vi "SetTrendPointProperties.vi"(8 "error in (no error)":errorcluster, 10 "map":T2, 11 "data set id":string) -> (0 "error out":errorcluster, 3 "properties":T1[](array[typedef]))   [LabVIEW 2017, in "IrDataEventCreator.lvlib"]
uses:
  <vilib>/addons/InsightCM/Devices/Shared/Ir/IrDataEventCreator/IrDataEventCreator.lvlib
  <vilib>/addons/PointValueMap/controls/PointMap.ctl
  <vilib>/addons/InsightCM/MessageBus/Base/controls/KeyValuePair.ctl
  <vilib>/addons/PointValueMap/subVIs/Point_Read_string.vi
  <vilib>/addons/PointValueMap/PointValueMap.lvlib
  <vilib>/addons/InsightCM/Utilities/PropertyHelpers/PropertyHelpers.lvlib
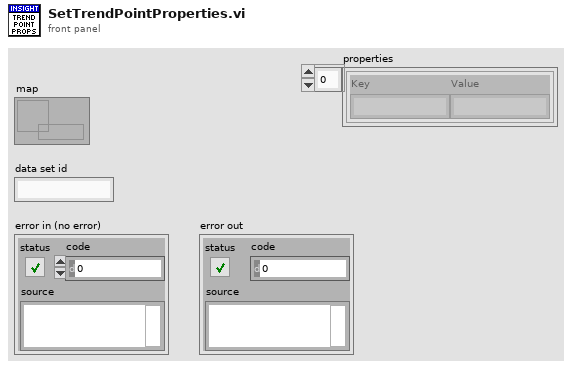
[diagram p1: front panel]
types:
  T1 = typedef "KeyValuePair.ctl" = cluster{"Key":string, "Value":string}
  T2 = typedef "PointValueMap.lvlib/PointMap.ctl" = refnum<data-value>
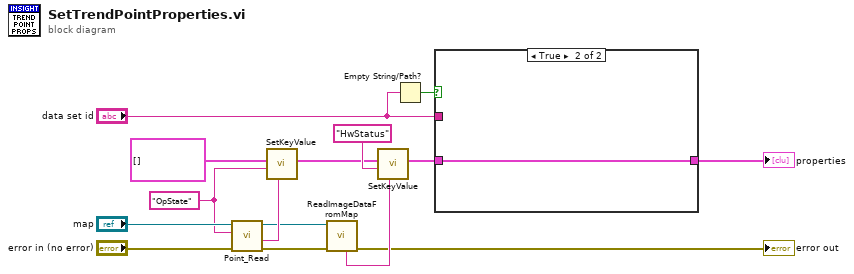
[diagram p0: block diagram]
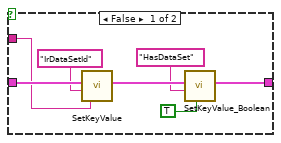
[diagram p2: hidden frame]
diagram:
  w6 = "OpState" ("Tag")
  n1 = call-poly <vilib>:"Point_Read.vi"("Error In"="error in (no error)", "Tag"=w6, "Map"="map") -> ("Error Out"=w3:errorcluster, "Value"=w5:string, "Map Out"=w4:T2)  [unwired: 3 in, 3 out]
  n2 = call <vilib>:"SetKeyValue.vi"("value"=w5, "key"=w6, "key value pairs"=T1[] [] ("props in")) -> ("key value pairs out"=w8:T1[])  [unwired: 8 in]
  n3 = call <vilib>:"ReadImageDataFromMap.vi"("map"=w4, "error in (no error)"=w3) -> ("error out"=→"error out":errorcluster, "image status"=w2:string)  [unwired: 3 in, 5 out]
  n4 = call <vilib>:"SetKeyValue.vi"("value"=w2, "key"="HwStatus", "key value pairs"=w8) -> ("key value pairs out"=w15:T1[])  [unwired: 8 in]
  n5 = Empty String/Path?(string/path="data set id") -> (empty?=w13:bool)
  n6 = case shown="True" w13 {
    tunnel: "data set id" -> [w21 _]
    tunnel: w15 -> [w22 w23]
    tunnel: [w18 w23] -> w11
    frame False {
      n7 = call <vilib>:"SetKeyValue.vi"("value"=w21, "key"="IrDataSetId", "key value pairs"=w22) -> ("key value pairs out"=w19:T1[])  [unwired: 8 in]
      n8 = call <vilib>:"SetKeyValue_Boolean.vi"("value"=TRUE, "key"="HasDataSet", "key value pairs"=w19) -> ("key value pairs out"=w18:T1[])  [unwired: 8 in]
    }
    frame True {
    }
  }
  "properties" <- w11
